vi "calculate.vi"(11 "data in":T2) -> (3 "data out":T2)   [LabVIEW 2020]
uses:
  Problem-21/Cluster_Monkey Data.ctl
  Problem-21/ENUM_Operator.ctl
panel:
  out "Operator":T1
  out "2":i64
  out "1":i64
  out "value":i64
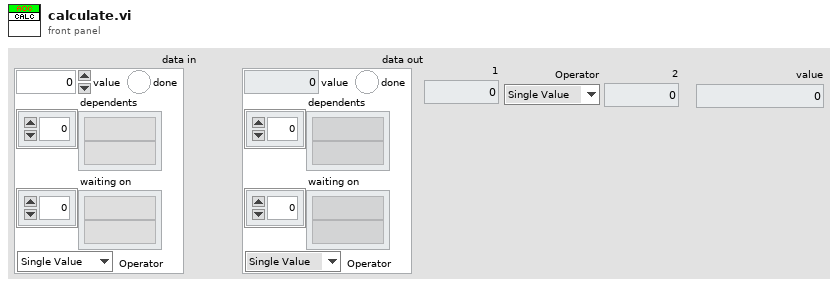
[diagram p1: front panel]
types:
  T1 = typedef "ENUM_Operator.ctl" = enum16{"Single Value", "Add", "Subtract", "Multiply", "Divide"}
  T2 = typedef "Cluster_Monkey Data.ctl" = cluster{"done":bool, "value":i64, "dependents":string[], "waiting on":string[], "Operator":T1}
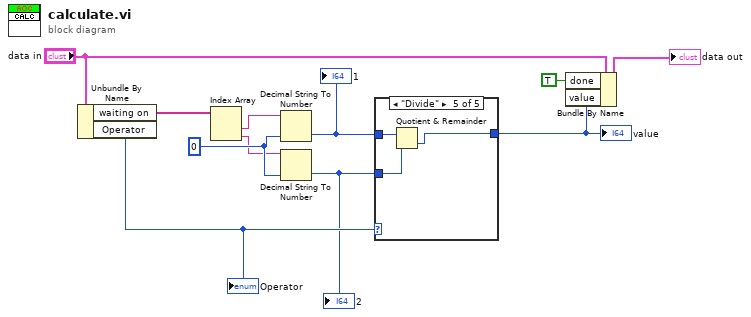
[diagram p0: block diagram]
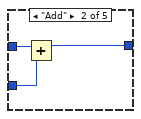
[diagram p3: hidden frame]
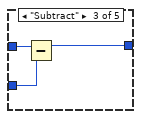
[diagram p4: hidden frame]
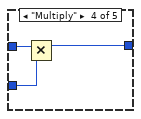
[diagram p5: hidden frame]
diagram:
  w5 = i64 0
  n1 = Unbundle By Name("data in") -> ("waiting on"=w7:string[], "Operator"=w8:T1)
  "Operator" <- w8
  n2 = Index Array(array=w7) -> (element #1=w4:string, element #2=w3:string)  [unwired: 2 in]
  n3 = Decimal String To Number(string=w4, default (0L)=w5) -> (number=w2:i64)  [unwired: 1 in, 1 out]
  "1" <- w2
  n4 = Decimal String To Number(string=w3, default (0L)=w5) -> (number=w1:i64)  [unwired: 1 in, 1 out]
  "2" <- w1
  n5 = case shown="\"Divide\"" w8 {
    tunnel: w2 -> [w12 w15 w18 w21 w24]
    tunnel: w1 -> [_ w14 w17 w20 w23]
    tunnel: [w12 w13 w16 w19 w22] -> w6
    frame "Single Value" {
    }
    frame "Add" {
      n6 = Add(x=w15, y=w14) -> (x+y=w13:i64)
    }
    frame "Subtract" {
      n7 = Subtract(x=w18, y=w17) -> (x-y=w16:i64)
    }
    frame "Multiply" {
      n8 = Multiply(x=w21, y=w20) -> (x*y=w19:i64)
    }
    frame "Divide" {
      n9 = Quotient & Remainder(x=w24, y=w23) -> (floor(x/y)=w22:i64)  [unwired: 1 out]
    }
  }
  "value" <- w6
  n10 = Bundle By Name(cluster="data in", "done"=TRUE, "value"=w6) -> (→"data out":T2)
